vi "Vision Research Phantom Series PhCon PhVideoPlay.vi"(0 "CN in":u32=1, 1 "CineNr":i32, 2 "pRng":T1, 3 "PlaySpeed":i32, 5 "Error In (no error)":errorcluster) -> (14 "CN out":u32=1, 19 "Error Out":errorcluster)   [LabVIEW 2013, in "VRI.lvlib"]
doc: "PhCon.dll\n\nPhVideoPlay\nHRESULT PhVideoPlay(UINT CN, int CineNr, PIMRANGE pRng, int PlaySpeed)\n\nParameters Description\nCN (in) Camera number.\nCineNr (in) Cine number. The cine has to be already recorded.\npRng (in) Range of images from the cine to play; if the pointer to the \n range is NULL this call changes only the playback speed to the \n value specified in the PlaySpeed parameter.\nPlaySpeed (in) Playback speed in milihertz (1000 means 1 frame per second).\n Negative speed means play backward.\nReturn HRESULT (0 = Ok)\nComments Plays back a clip from the specified cine to the camera video\n out.\n If CineNr <1 the video will show preview images.\n When pRng->Cnt = 0 or PlaySpeed = 0 it will continuously\n show the pRng->FirstImage (Pause Mode). Using this feature,\n you can implement Step forward, backward and browse with a\n trackbar in your client software.\n If pRng->Cnt !=0 it will playback the specified range of\n images in the camera, forward or backward depending on the\n sign of the PlaySpeed."
uses:
  VRI.lvlib
  _Type Defs/PHCon IMRANGE.ctl
  Phantom DLLs/PhCon.Dll
panel:
  # "For instructions on the use of this VI, press Ctrl+H to display the help window and move the mouse over the icon, controls, and indicators"
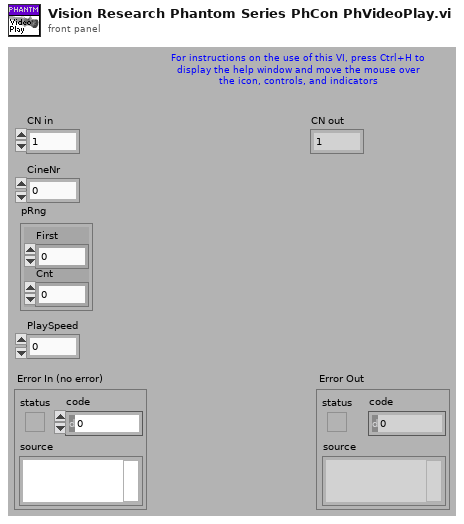
[diagram p1: front panel]
types:
  T1 = typedef "VRI.lvlib/PHCon IMRANGE.ctl" = cluster{"First":i32, "Cnt":u32}
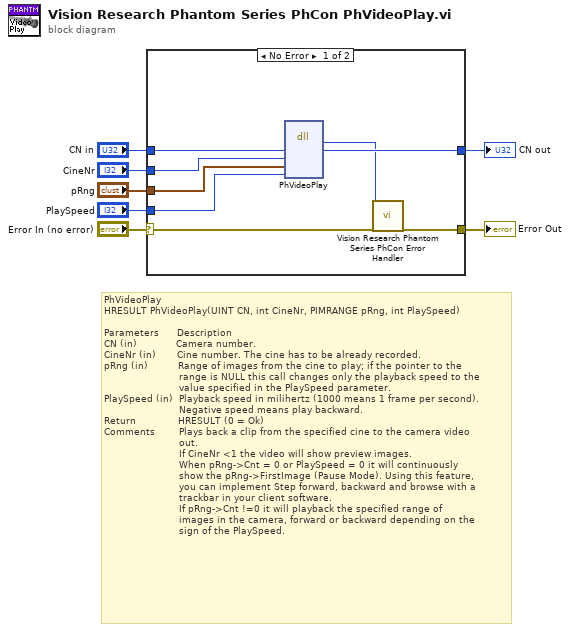
[diagram p0: block diagram]
diagram:
  # "PhVideoPlay\nHRESULT PhVideoPlay(UINT CN, int CineNr, PIMRANGE pRng, int PlaySpeed)\n\nParameters      Description\nCN (in)             Camera number.\nCineNr (in)       Cine number. The cine has to be already recorded.\npRng (in)          Range of images from the cine to play; if the pointer to the \n                         range is NULL this call changes only the playback speed to the \n                         value specified in the PlaySpeed parameter.\nPlaySpeed (in)  Playback speed in milihertz (1000 means 1 frame per second).\n                         Negative speed means play backward.\nReturn              HRESULT (0 = Ok)\nComments        Plays back a clip from the specified cine to the camera video\n                         out.\n                         If CineNr <1 the video will show preview images.\n                         When pRng->Cnt = 0 or PlaySpeed = 0 it will continuously\n                         show the pRng->FirstImage (Pause Mode). Using this feature,\n                         you can implement Step forward, backward and browse with a\n                         trackbar in your client software.\n                         If pRng->Cnt !=0 it will playback the specified range of\n                         images in the camera, forward or backward depending on the\n                         sign of the PlaySpeed."
  n1 = case shown="No Error" "Error In (no error)" {
    selector: "Error In (no error)" -> [w15 w17]
    tunnel: [w14 w17] -> w6
    tunnel: "CN in" -> [w13 w16]
    tunnel: [w12 w16] -> w4
    tunnel: "CineNr" -> [w11 _]
    tunnel: "pRng" -> [w10 _]
    tunnel: "PlaySpeed" -> [w9 _]
    frame No Error {
      n2 = dll-call lib="C:/Projects/SDK/64-bit/Vision Research Phantom Series Labview Driver/Phantom DLLs/PhCon.dll" fn="PhVideoPlay"("CN"=w13, "CineNr"=w11, "pRng"=w10, "PlaySpeed"=w9) -> ("HRESULT"=w8:i32, "CN"=w12:u32)  [unwired: 6 in, 2 out]
      n3 = call "Vision Research Phantom Series PhCon Error Handler.vi"("ErrNo"=w8, "Error In (no error)"=w15) -> ("Error Out"=w14:errorcluster)  [unwired: 17 out]
    }
    frame Error {
    }
  }
  "Error Out" <- w6
  "CN out" <- w4
